vi "Run Step.vi"(8 "error in (no error)":errorcluster, 9 "result allocation":T1, 10 "parameters":T1, 11 "Wait On Integer Step in":refnum<class "Wait On Integer Step.lvclass">) -> (0 "error out":errorcluster, 1 "results":T1, 2 "parameter allocation":T1, 3 "Wait On Integer Step out":refnum<class "Wait On Integer Step.lvclass">)   [LabVIEW 2015, in "Wait On Integer Step.lvclass"]
uses:
  Wait On Integer Step.lvclass
  <vilib>/NI/Tag Bus/table/data table.ctl
  Wait On Integer Step.lvclass/Wait On Integer Step.ctl
  <vilib>/NI/Tag Bus/table/data polymorphs/read one/read U32.vi
  Write Timer Value (ms).vi
  <vilib>/NI/Tag Bus/table/data table.lvlib
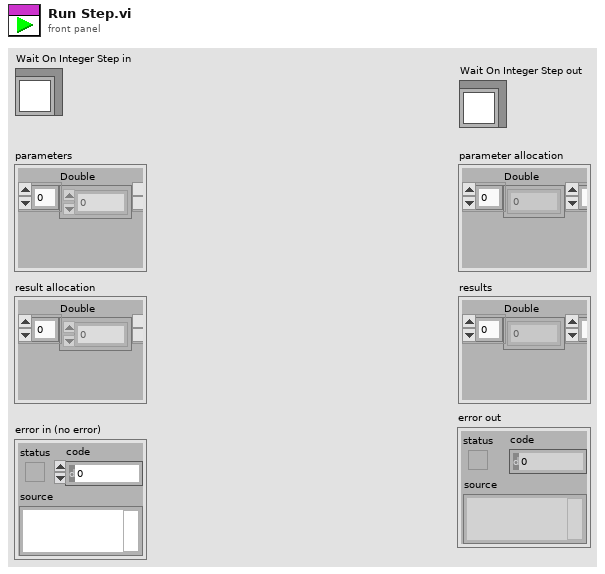
[diagram p1: front panel]
types:
  T1 = typedef "tag bus.lvlib/data table.lvlib/data table.ctl" = cluster{"Double":dbl[], "Single":sgl[], "I64":i64[], "I32":i32[], "I16":i16[], "I8":i8[], "U64":u64[], "U32":u32[], "U16":u16[], "U8":u8[], "Boolean":bool[], "String":string[], "Array of Double":cluster{"DBL Array":dbl[]}[], "Array of Single":cluster{"SGL Array":sgl[]}[], "Array of I64":cluster{"I64 Array":i64[]}[], "Array of I32":cluster{"I32 Array":i32[]}[], "Array of I16":cluster{"I16 Array":i16[]}[], "Array of I8":cluster{"I8 Array":i8[]}[], "Array of U64":cluster{"U64 Array":u64[]}[], "Array of U32":cluster{"U32 Array":u32[]}[], "Array of U16":cluster{"U16 Array":u16[]}[], "Array of U8":cluster{"U8 Array":u8[]}[], "Array of Boolean":cluster{"Boolean Array":bool[]}[], "Array of String":cluster{"String Array":string[]}[]}
  T2 = typedef "Step.lvclass/StepState.ctl" = cluster{"Step State":T3, "Flow Control":T4, "Jump Index":i32, "Done":bool}
  T3 = typedef "Step.lvclass/Step Status.ctl" = enum16{"Start", "Passed", "Failed", "Error", "Done", "Terminated", "Skipped", "Running"}
  T4 = typedef "Step.lvclass/Step Flow Control.ctl" = enum16{"Next Step", "Jump"}
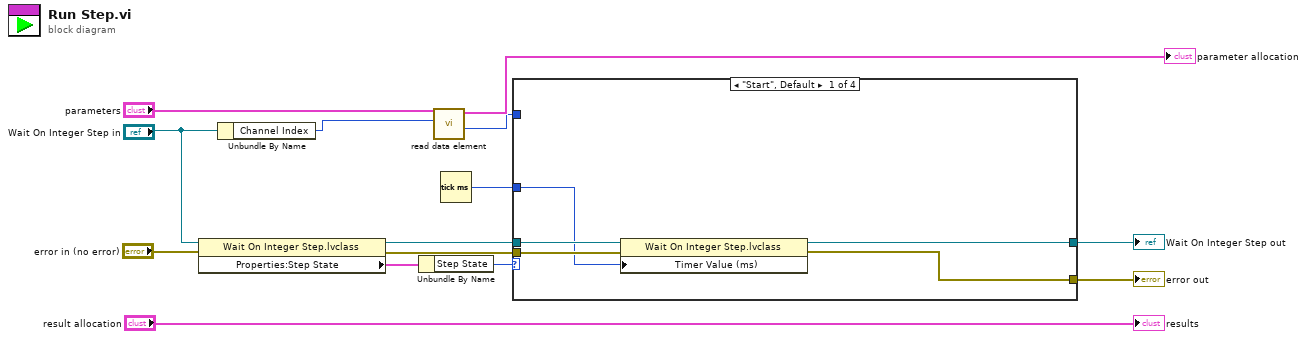
[diagram p0: block diagram]
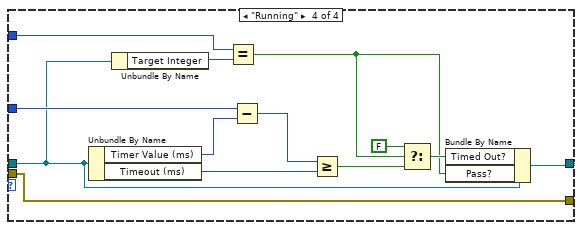
[diagram p4: hidden frame]
diagram:
  n1 = property class="Wait On Integer Step.lvclass"(reference="Wait On Integer Step in", error in="error in (no error)") -> (reference out=w12:refnum<class "Wait On Integer Step.lvclass">, error out=w11:errorcluster, "Properties:Step State"=w14:T2)
  n2 = Unbundle By Name("Wait On Integer Step in") -> ("Channel Index"=w9:i32)
  n3 = Unbundle By Name(w14) -> ("Step State"=w13:T3)
  n4 = call-poly <vilib>:"read data element.vi"("index"=w9, "data table in"="parameters") -> ("value"=w1:u32, "data table out"=→"parameter allocation":T1)  [unwired: 8 in]
  n5 = Tick Count (ms)() -> (millisecond timer value=w10:u32)
  n6 = case shown="\"Start\", Default" w13 {
    tunnel: w12 -> [w18 w20 w22 w27]
    tunnel: w11 -> [w19 w21 w23 w31]
    tunnel: [w17 w20 w22 w32] -> w2
    tunnel: w10 -> [w16 _ _ w35]
    tunnel: [w15 w21 w23 w31] -> w3
    tunnel: w1 -> [_ _ _ w25]
    frame "Start", Default {
      n7 = property class="Wait On Integer Step.lvclass"(reference=w18, error in=w19, "Timer Value (ms)"=w16) -> (reference out=w17:refnum<class "Wait On Integer Step.lvclass">, error out=w15:errorcluster)
    }
    frame "Skipped" {
    }
    frame "Error" {
    }
    frame "Running" {
      n8 = Unbundle By Name(w27) -> ("Timer Value (ms)"=w36:i32, "Timeout (ms)"=w33:i32)
      n9 = Unbundle By Name(w27) -> ("Target Integer"=w26:u32)
      n10 = Equal?(x=w25, y=w26) -> (x = y?=w24:bool)
      n11 = Subtract(x=w35, y=w36) -> (x-y=w34:u32)
      n12 = Greater Or Equal?(x=w34, y=w33) -> (x >= y?=w29:bool)
      n13 = Select(t=FALSE ("value"), s=w24, f=w29) -> (s? t:f=w28:bool)
      n14 = Bundle By Name(cluster=w27, "Timed Out?"=w28, "Pass?"=w24) -> (w32:refnum<class "Wait On Integer Step.lvclass">)
    }
  }
  "error out" <- w3
  "Wait On Integer Step out" <- w2
  "results" <- "result allocation"
